vi "test Delete Endpoint String From Valid Alias.vi"(8 "error in (no error)":errorcluster, 11 "TestCase in":refnum<class "Routing and Faulting Aliases Unit Tests.lvclass">) -> (0 "error out":errorcluster, 3 "TestCase out":refnum<class "Routing and Faulting Aliases Unit Tests.lvclass">)   [LabVIEW 2020, in "Routing and Faulting Aliases Unit Tests.lvclass"]
uses:
  Routing and Faulting Aliases Unit Tests.lvclass
  System Explorer/Alias.ctl
  System Explorer/Endpoint.ctl
  Shared/Alias Endpoint.ctl
  Shared/Alias Mapping.ctl
  Routing and Faulting Aliases Unit Tests.lvclass/Routing and Faulting Aliases Unit Tests.ctl
  <vilib>/addons/_JKI Toolkits/VI Tester/TestCase.llb/TestCase.lvclass
  System Explorer/Routing and Faulting System Explorer.lvlib
  Scripting/Routing and Faulting Scripting.lvlib
  Shared/Routing and Faulting Shared.lvlib
  C:/Program Files (x86)/National Instruments/LabVIEW 2020/vi.lib/addons/_JKI Toolkits/VI Tester/TestCase.llb/TestCase.lvclass
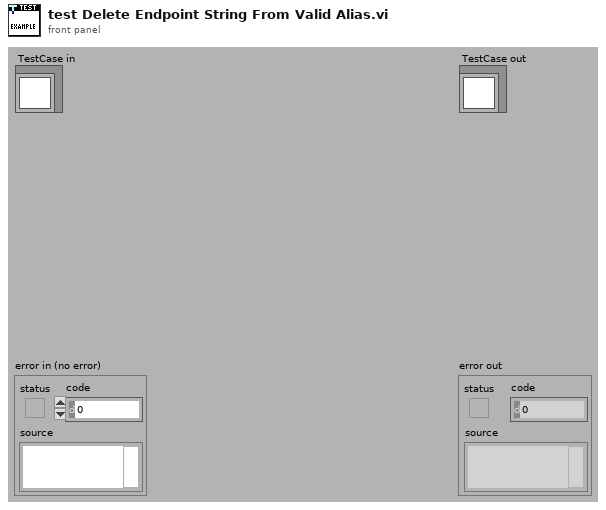
[diagram p1: front panel]
types:
  T1 = typedef "Routing and Faulting Shared.lvlib/Alias Endpoint.ctl" = cluster{"Module Path":string, "Endpoint":string}
  T2 = typedef "Routing and Faulting Shared.lvlib/Alias Mapping.ctl" = cluster{"Alias":string, "Endpoint":T1}
  T3 = typedef "Routing and Faulting System Explorer.lvlib/Endpoint.ctl" = string
  T4 = typedef "Routing and Faulting System Explorer.lvlib/Alias.ctl" = cluster{"Endpoint":T3, "Alias":string, "Remove":bool}
  T5 = typedef "Custom Device API.lvlib/Custom Device Item Ref.ctl" = u64
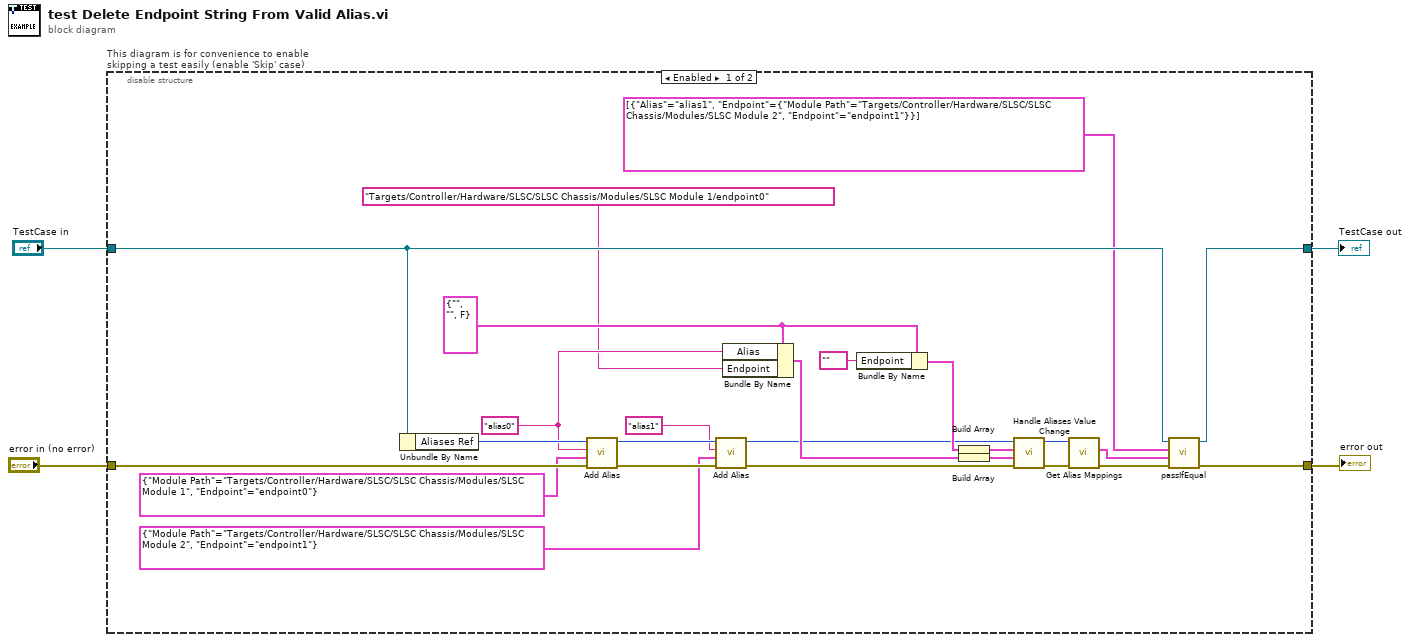
[diagram p0: block diagram]
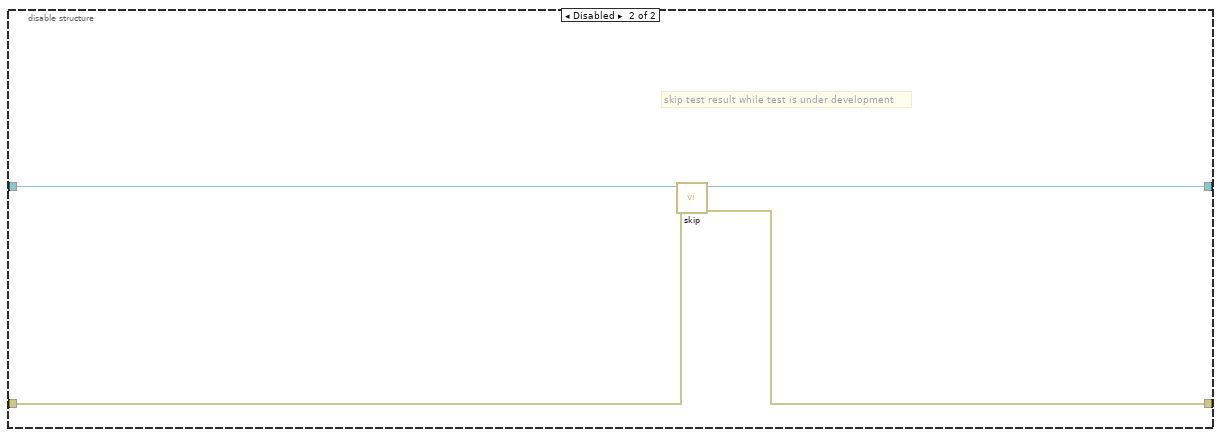
[diagram p2: hidden frame]
diagram:
  n1 = disable-structure "This diagram is for convenience to enable skipping a test easily (enable 'Skip' case)" shown="Enabled" {
    disable-tunnel: "TestCase in" -> [w25 w33]
    disable-tunnel: [w24 w31] -> w1
    disable-tunnel: [w26 w32] -> w3
    disable-tunnel: "error in (no error)" -> [w22 w30]
    frame Enabled {
      w20 = T4 {"Endpoint"="", "Alias"="", "Remove"=FALSE} ("Alias")
      w21 = "alias0" ("Alias")
      n2 = Unbundle By Name(w25) -> ("Aliases Ref"=w23:T5)
      n3 = call "Add Alias.vi"("error in"=w22, "endpoint"=T1 {"Module Path"="Targets/Controller/Hardware/SLSC/SLSC Chassis/Modules/SLSC Module 1", "Endpoint"="endpoint0"} ("Endpoint"), "alias"=w21, "endpoint aliases in"=w23) -> ("error out"=w14:errorcluster, "endpoint aliases out"=w13:T5)  [unwired: 6 in]
      n4 = call "Add Alias.vi"("error in"=w14, "endpoint"=T1 {"Module Path"="Targets/Controller/Hardware/SLSC/SLSC Chassis/Modules/SLSC Module 2", "Endpoint"="endpoint1"} ("Endpoint"), "alias"="alias1" ("Alias"), "endpoint aliases in"=w13) -> ("error out"=w11:errorcluster, "endpoint aliases out"=w10:T5)  [unwired: 6 in]
      n5 = Bundle By Name(cluster=w20, "Alias"=w21, "Endpoint"=T3 "Targets/Controller/Hardware/SLSC/SLSC Chassis/Modules/SLSC Module 1/endpoint0") -> (w17:T4)
      n6 = Bundle By Name(cluster=w20, "Endpoint"=T3 "") -> (w18:T4)
      n7 = Build Array(w18) -> (w16:T4[])
      n8 = Build Array(w17) -> (w15:T4[])
      n9 = call "Handle Aliases Value Change.vi"("error in (no error)"=w11, "OldVal"=w15, "NewVal"=w16, "Aliases Ref in"=w10) -> ("error out"=w29:errorcluster, "Aliases Ref out"=w28:T5)  [unwired: 4 in, 2 out]
      n10 = call "Get Alias Mappings.vi"("error in"=w29, "endpoint aliases in"=w28) -> ("error out"=w27:errorcluster, "alias mappings"=w9:T2[])  [unwired: 7 in, 1 out]
      n11 = call-dynamic "passIfEqual.vi"("error in (no error)"=w27, "y"=w9, "x"=T2[] [{"Alias"="alias1", "Endpoint"={"Module Path"="Targets/Controller/Hardware/SLSC/SLSC Chassis/Modules/SLSC Module 2", "Endpoint"="endpoint1"}}] ("Alias Mappings"), "TestCase in"=w25) -> ("error out"=w26:errorcluster, "TestCase out"=w24:refnum<class "Routing and Faulting Aliases Unit Tests.lvclass">)  [unwired: 6 in]
    }
    frame Disabled {
      # "skip test result while test is under development"
      n12 = call <vilib>:"skip.vi"("error in (no error)"=w30, "TestCase in"=w33) -> ("error out"=w32:errorcluster, "TestCase out"=w31:refnum<class "Routing and Faulting Aliases Unit Tests.lvclass">)  [unwired: 8 in]
    }
  }
  "error out" <- w3
  "TestCase out" <- w1
